vi "Open Report File.vi"(8 "error in (no error)":errorcluster, 10 "Report Path":path, 11 "XML Report In":refnum<class "XML Report.lvclass">) -> (0 "error out":errorcluster, 3 "XML Report Out":refnum<class "XML Report.lvclass">)   [LabVIEW 2020, in "Reports.lvlib" / "XML Report.lvclass"]
uses:
  XML Report.lvclass
  Core/Result/Result.ctl
  Core/Result/Status.ctl
  Core/Result/Type.ctl
  XML Report.lvclass/XML Report.ctl
  <vilib>/xml/NI_XML.lvlib
  <resource>/objmgr/DOMUserDefRef.rc
  Core/Result/Result.lvlib
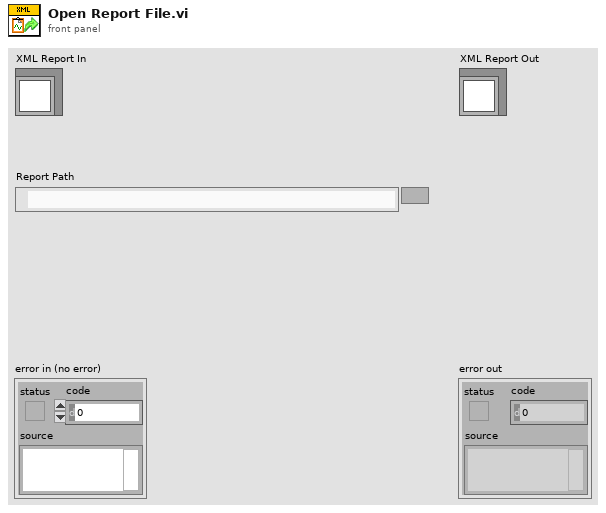
[diagram p1: front panel]
types:
  T1 = typedef "Result.lvlib/Result.ctl" = cluster{"Name":string, "Message":string, "Description":string, "Status":T2, "Result Type":T3, "Execution Time":dbl}
  T2 = typedef "Result.lvlib/Status.ctl" = enum16{"", "Passed", "Failed", "Error", "Skipped", "Setup Error", "Broken", "Teardown Error"}
  T3 = typedef "Result.lvlib/Type.ctl" = enum16{"Method", "Case", "Suite", "Pass", "Fail", "Skip", "Pass if", "Fail if", "Pass if Error", "Fail if Error", "Pass if Equal", "Fail if Equal"}
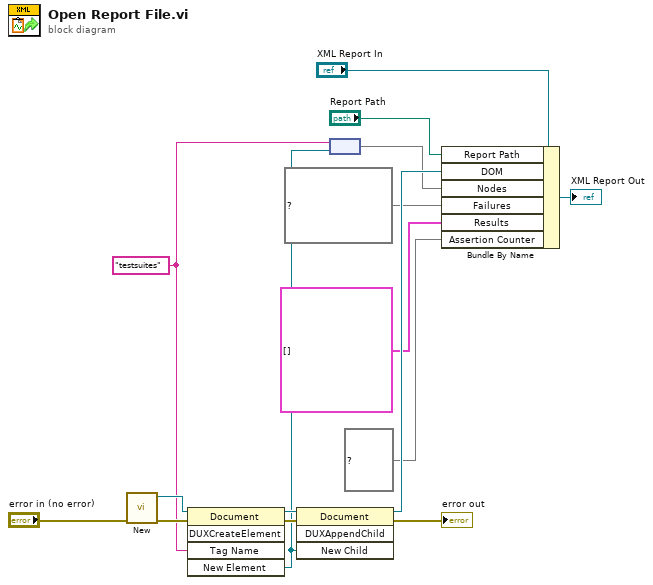
[diagram p0: block diagram]
diagram:
  w6 = "testsuites" ("Tag Name")
  n1 = call <vilib>:"New.vi"("error in (no error)"="error in (no error)") -> ("error out"=w9:errorcluster, "DOM document out"=w12:refnum<k20>)  [unwired: 7 in]
  n2 = invoke class="Document" method="DUXCreateElement"(reference=w12, error in=w9, "Tag Name"=w6) -> (reference out=w11:refnum<k20>, error out=w10:errorcluster, "New Element"=w5:refnum<k20>)  [unwired: 2 in, 2 out]
  n3 = invoke class="Document" method="DUXAppendChild"(reference=w11, error in=w10, "New Child"=w5) -> (reference out=w7:refnum<k20>, error out=→"error out":errorcluster)  [unwired: 1 in, 2 out]
  n4 = node(w6, w5) -> (w4:map{string, refnum<k20>})
  n5 = Bundle By Name(cluster="XML Report In", "Report Path"="Report Path", "DOM"=w7, "Nodes"=w4, "Failures"=map{string, refnum<k20>[]} {}, "Results"=T1[] [], "Assertion Counter"=map{string, i32} {}) -> (→"XML Report Out":refnum<class "XML Report.lvclass">)
